vi "ReScalePlots.vi"(9 "View Type":u16, 10 "plot out":refnum<vi>, 11 "WaveformGraph in":refnum<vi>) -> ()   [LabVIEW 2024]
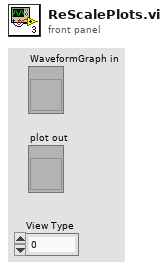
[diagram p1: front panel]
types:
  T1 = typedef "LVRangeTypeDef.ctl" = cluster{"Minimum":dbl, "Maximum":dbl, "Increment":dbl, "Minor Increment":dbl, "Start":dbl}
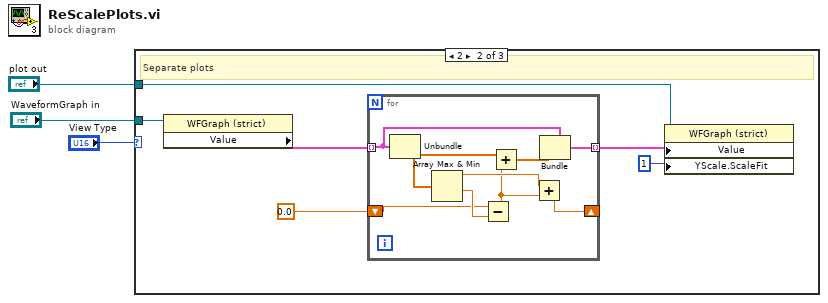
[diagram p0: block diagram]
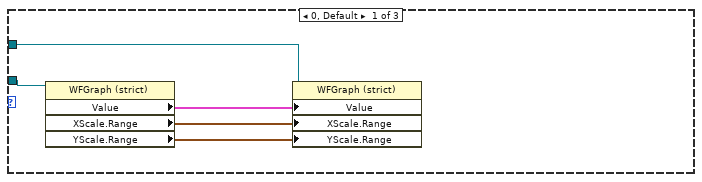
[diagram p2: hidden frame]
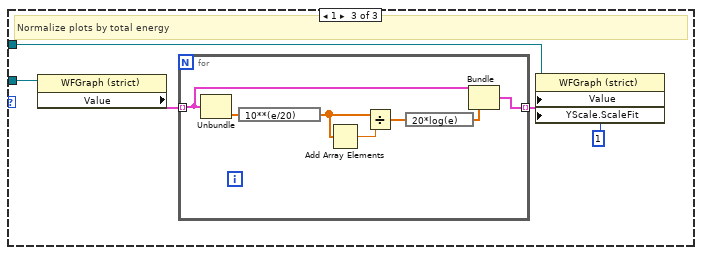
[diagram p3: hidden frame]
diagram:
  n1 = case shown="2" "View Type" {
    tunnel: "WaveformGraph in" -> [w7 w14 w28]
    tunnel: "plot out" -> [w8 w10 w25]
    frame 0, Default {
      n2 = property class="WFGraph (strict)"(reference=w7) -> ("Value"=w6:cluster{dbl, "dt":dbl, "Y":dbl[]}[], "XScale.Range"=w5:T1, "YScale.Range"=w4:T1)  [unwired: 1 in, 2 out]
      n3 = property class="WFGraph (strict)"(reference=w8, "Value"=w6, "XScale.Range"=w5, "YScale.Range"=w4) -> ()  [unwired: 1 in, 2 out]
    }
    frame 2 {
      # "Separate plots"
      n4 = property class="WFGraph (strict)"(reference=w14) -> ("Value"=w13:cluster{dbl, "dt":dbl, "Y":dbl[]}[])  [unwired: 1 in, 2 out]
      n5 = for {
        tunnel: w13 -> [w19] mode=indexing
        shift-right: [w15] -> _
        shift-left: 0.0 -> [w21]
        tunnel: [w18] -> w11 mode=indexing
        n6 = Unbundle(w19) -> ("Y"=w22:dbl[])  [unwired: 2 out]
        n7 = Array Max & Min(array=w22) -> (max value=w17:dbl, min value=w23:dbl)  [unwired: 2 out]
        n8 = Subtract(x=w21, y=w23) -> (x-y=w16:dbl)
        n9 = Add(x=w22, y=w16) -> (x+y=w20:dbl[])
        n10 = Add(x=w17, y=w16) -> (x+y=w15:dbl)
        n11 = Bundle(cluster=w19, "Y"=w20) -> (w18:cluster{dbl, "dt":dbl, "Y":dbl[]})  [unwired: 2 in]
      }
      n12 = property class="WFGraph (strict)"(reference=w10, "Value"=w11, "YScale.ScaleFit"=u8 1 ("Y Scale.Scale Fit")) -> ()  [unwired: 1 in, 2 out]
    }
    frame 1 {
      # "Normalize plots by total energy"
      n13 = property class="WFGraph (strict)"(reference=w28) -> ("Value"=w27:cluster{dbl, "dt":dbl, "Y":dbl[]}[])  [unwired: 1 in, 2 out]
      n14 = for {
        tunnel: w27 -> [w35] mode=indexing
        tunnel: [w34] -> w26 mode=indexing
        n15 = Unbundle(w35) -> ("Y"=w32:dbl[])  [unwired: 2 out]
        n16 = expression code="10**(e/20)"(w32) -> (w30:dbl[])
        n17 = Add Array Elements(numeric array=w30) -> (sum=w33:dbl)
        n18 = Divide(x=w30, y=w33) -> (x/y=w31:dbl[])
        n19 = expression code="20*log(e)"(w31) -> (w29:dbl[])
        n20 = Bundle(cluster=w35, "Y"=w29) -> (w34:cluster{dbl, "dt":dbl, "Y":dbl[]})  [unwired: 2 in]
      }
      n21 = property class="WFGraph (strict)"(reference=w25, "Value"=w26, "YScale.ScaleFit"=u8 1 ("Y Scale.Scale Fit")) -> ()  [unwired: 1 in, 2 out]
    }
  }
